vi "Connect.vi"(8 "error in (no error)":errorcluster, 10 "Device ID":i32) -> (0 "error out":errorcluster, 3 "midi out out":refnum<class "midi out.lvclass">)   [LabVIEW 2020, in "midi out.lvclass"]
uses:
  midi out.lvclass
  midi out.lvclass/midi out.ctl
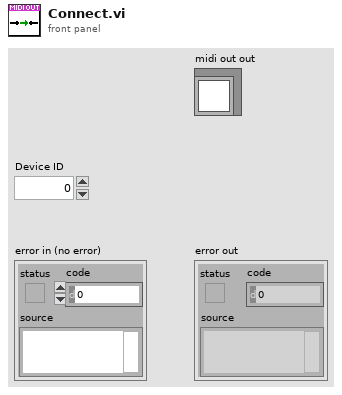
[diagram p1: front panel]
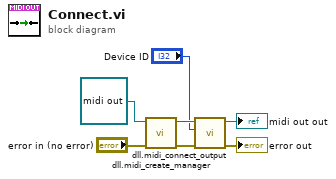
[diagram p0: block diagram]
diagram:
  n1 = call "dll.midi_create_manager.vi"("error in (no error)"="error in (no error)", "midi out in"=refnum<class "midi out.lvclass"> refnum) -> ("error out"=w5:errorcluster, "midi out"=w6:refnum<class "midi out.lvclass">)  [unwired: 8 in]
  n2 = call "dll.midi_connect_output.vi"("error in (no error)"=w5, "device_index"="Device ID", "midi out in"=w6) -> ("error out"=→"error out":errorcluster, "midi out"=→"midi out out":refnum<class "midi out.lvclass">)  [unwired: 7 in]
